vi "Clean Up String SubVI.vi"(11 "String from OCR":string[](array[string])) -> (3 "Cleaned Up String":string[](array[string]))   [LabVIEW 2014]
doc: "This subVI takes out all the empty or less than 3 character strings and cleans up the input array."
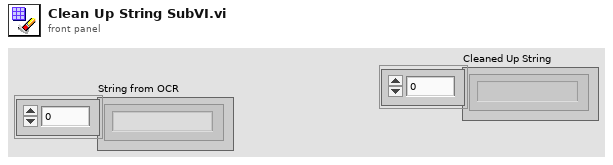
[diagram p1: front panel]
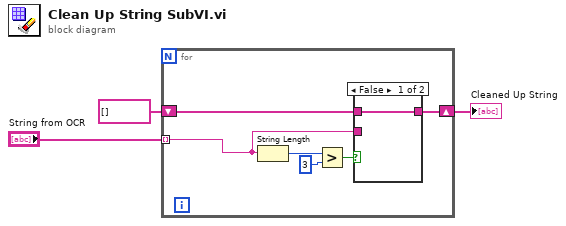
[diagram p0: block diagram]
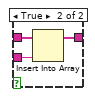
[diagram p2: hidden frame]
diagram:
  n1 = for {
    tunnel: "String from OCR" -> [w4] mode=indexing
    shift-right: [w5] -> w1
    shift-left: string[] [] -> [w6]
    n2 = String Length(string=w4) -> (length=w9:i32)
    n3 = Greater?(x=w9, y=3) -> (0:w7:bool)
    n4 = case shown="False" w7 {
      tunnel: w6 -> [w10 w13]
      tunnel: w4 -> [_ w12]
      tunnel: [w10 w11] -> w5
      frame False {
      }
      frame True {
        n5 = Insert Into Array(array=w13, new element=w12) -> (w11:string[])  [unwired: 1 in]
      }
    }
  }
  "Cleaned Up String" <- w1
